vi "InsertSampleSet.vi"(8 "error in":errorcluster, 11 "SampleSet":T1) -> (0 "error out":errorcluster)   [LabVIEW 2014, in "Sample.lvlib"]
uses:
  <vilib>/addons/database/Connection.llb/DB Tools Open Connec (String).vi
  <vilib>/addons/database/Connection.llb/Conn Execute.vi
  <vilib>/addons/database/Recordset.llb/Rec Destroy - Connection.vi
  Sample/Sample.lvlib
  <vilib>/addons/database/NI_Database_API.lvlib
  DataBase.lvlib
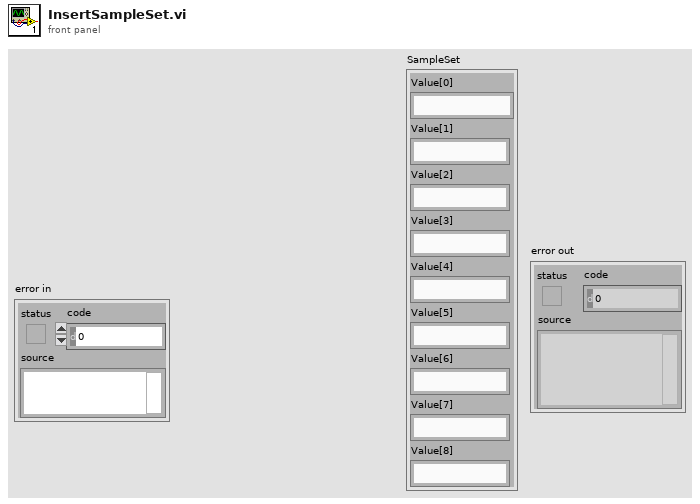
[diagram p1: front panel]
types:
  T1 = cluster{"Value[0]":string, "Value[1]":string, "Value[2]":string, "Value[3]":string, "Value[4]":string, "Value[5]":string, "Value[6]":string, "Value[7]":string, "Value[8]":string}
  T2 = typedef "NI_Database_API.lvlib/Conn ObjectReference.ctl" = refnum<k1>
  T3 = typedef "NI_Database_API.lvlib/Rec ObjectReference.ctl" = refnum<k1>
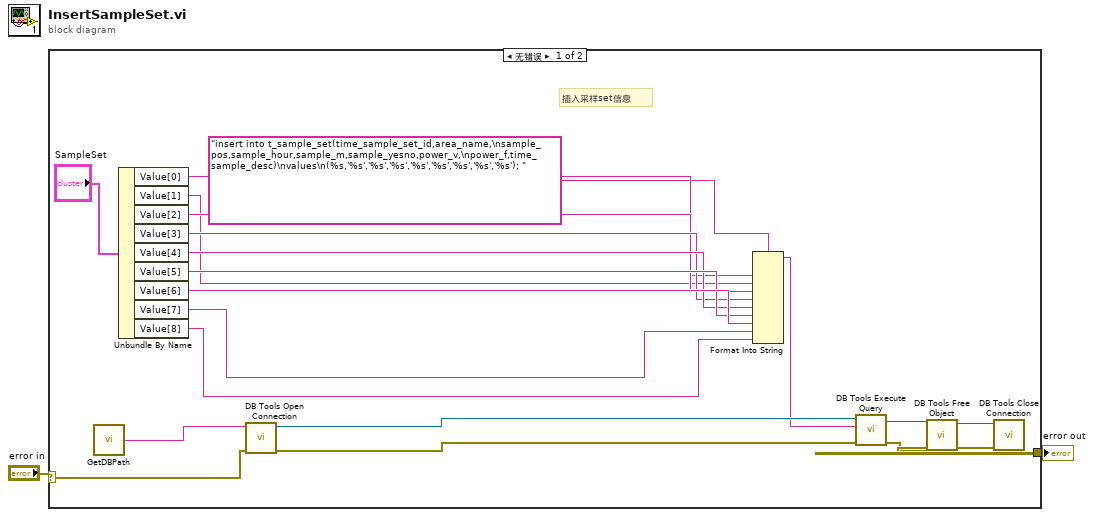
[diagram p0: block diagram]
diagram:
  n1 = case shown="无错误" "error in" {
    selector: "error in" -> [w19 w24]
    tunnel: [w18 w24] -> w1
    frame No Error {
      # "插入采样set信息"
      n2 = call "GetDBPath.vi"() -> ("Connection"=w17:string)  [unwired: 1 in]
      n3 = Unbundle By Name("SampleSet") -> ("Value[0]"=w6:string, "Value[1]"=w7:string, "Value[2]"=w8:string, "Value[3]"=w9:string, "Value[4]"=w10:string, "Value[5]"=w11:string, "Value[6]"=w12:string, "Value[7]"=w13:string, "Value[8]"=w14:string)
      n4 = call-poly <vilib>:"DB Tools Open Connection.vi"("error in (no error)"=w19, "connection information"=w17) -> ("error out"=w22:errorcluster, "connection reference"=w23:T2)  [unwired: 6 in]
      n5 = Format Into String(format string="insert into t_sample_set(time_sample_set_id,area_name,\nsample_pos,sample_hour,sample_m,sample_yesno,power_v,\npower_f,time_sample_desc)\nvalues\n(%s,'%s','%s','%s','%s','%s','%s','%s','%s'); ", w6, w7, w8, w9, w10, w11, w12, w13, w14) -> (resulting string=w3:string)  [unwired: 2 in, 1 out]
      n6 = call-poly <vilib>:"DB Tools Execute Query.vi"("error in (no error)"=w22, "SQL query"=w3, "connection reference"=w23) -> ("error out"=w15:errorcluster, "recordset reference"=w16:T3)  [unwired: 5 in]
      n7 = call-poly <vilib>:"DB Tools Free Object.vi"("error in (no error)"=w15, "recordset reference"=w16) -> ("error out"=w21:errorcluster, "connection reference"=w20:T2)  [unwired: 8 in]
      n8 = call <vilib>:"DB Tools Close Connection.vi"("error in (no error)"=w21, "connection reference"=w20) -> ("error out"=w18:errorcluster)  [unwired: 5 in]
    }
    frame Error {
    }
  }
  "error out" <- w1
